vi "TP_UI.vi"() -> ()   [LabVIEW 2012]
uses:
  Global Variants/TP_GV_UI_Ref.vi
panel:
  in  "Text Ring":u16(ring)
  in  "error in":errorcluster
  in  "OK Button":bool
  out "String":string
  in  "Stop Button":bool
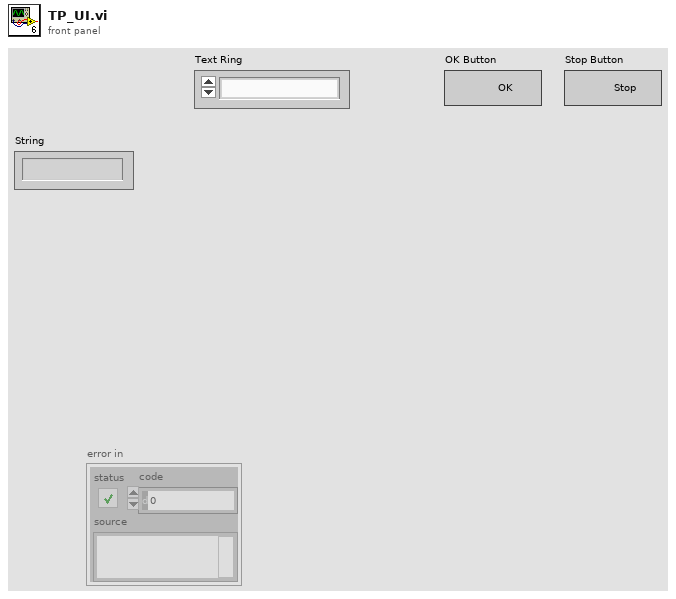
[diagram p1: front panel]
types:
  T1 = enum16{"Create Queue", "Get Queue", "Destory Queue"}
  T2 = enum16{"Create Queue", "Get Queue", "Destory Queue", "Destory all Queue"}
  T3 = cluster{"This VI":refnum<vi>, "String":refnum<vi>, "OK Button":refnum<vi>, "Stop Button":refnum<vi>, "Text Ring":refnum<vi>}
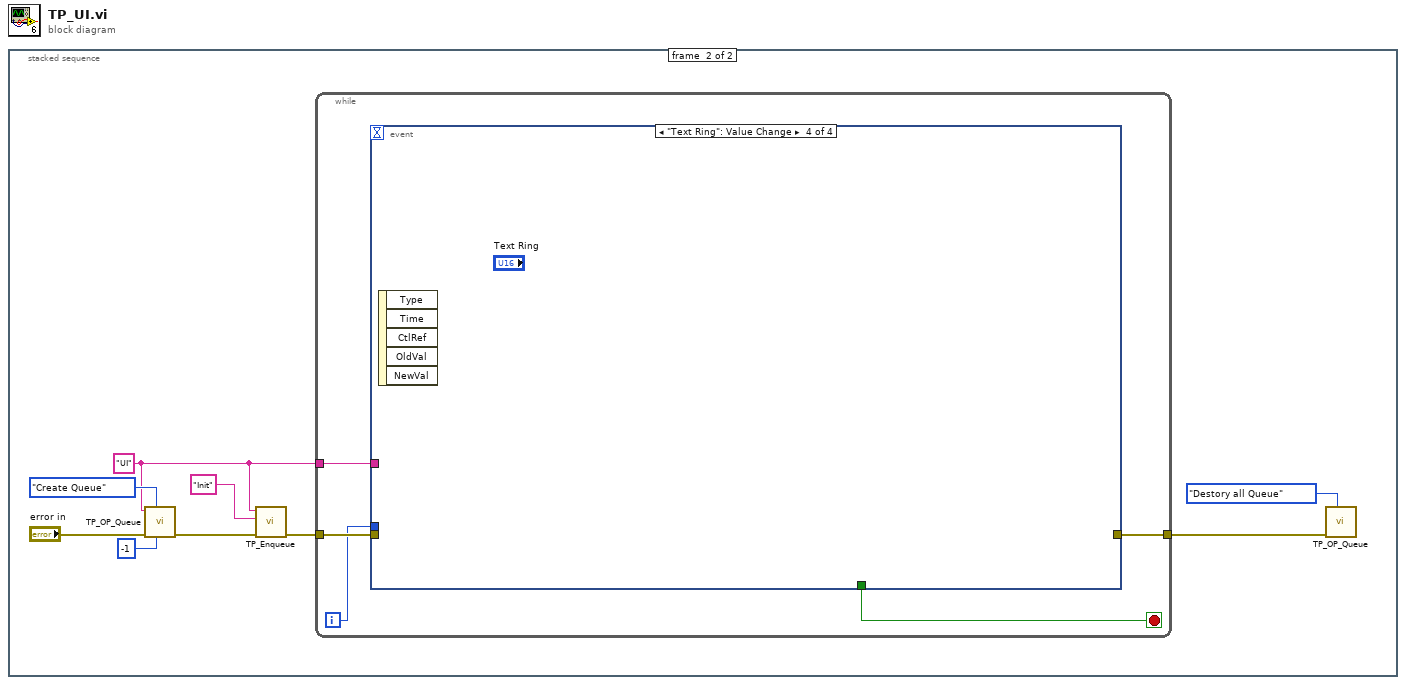
[diagram p0: block diagram]
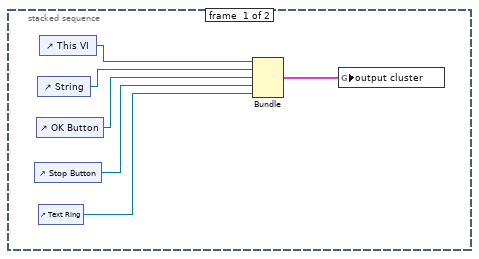
[diagram p2: hidden frame]
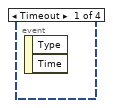
[diagram p3: hidden frame]
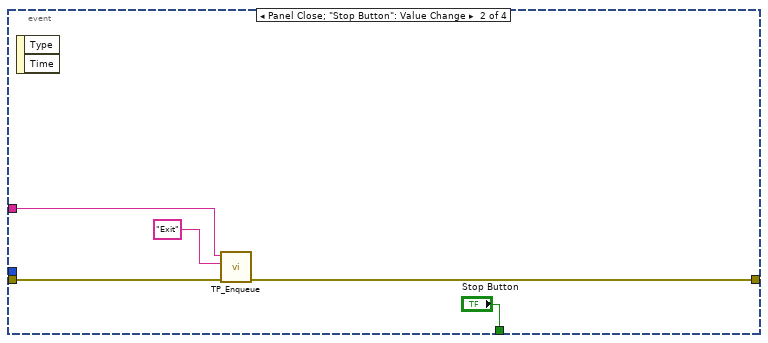
[diagram p4: hidden frame]
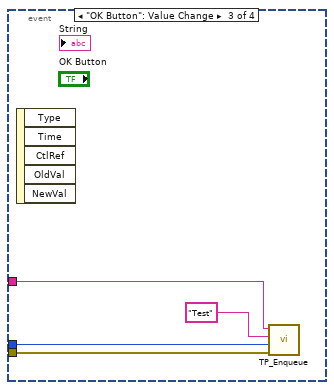
[diagram p5: hidden frame]
diagram:
  n1 = stacked-sequence {
    frame #0 {
      n2 = control-ref of="Stop Button"() -> (w3:refnum<vi>)
      n3 = control-ref of="OK Button"() -> (w4:refnum<vi>)
      n4 = control-ref of="String"() -> (w5:refnum<vi>)
      n5 = control-ref of="Text Ring"() -> (w1:refnum<vi>)
      n6 = control-ref of="This VI"() -> (w6:refnum<vi>)
      n7 = Bundle("This VI"=w6, "String"=w5, "OK Button"=w4, "Stop Button"=w3, "Text Ring"=w1) -> (w2:T3)  [unwired: 1 in]
      n8 = global write "TP_GV_UI_Ref.vi" "output cluster"(w2) -> ()
    }
    frame #1 {
      w8 = "UI" ("name (unnamed)")
      n9 = call "TP_OP_Queue.vi"("max queue size (-1, unlimited)"=-1, "OP_Queue (get queue)"=T1."Create Queue", "error in"="error in", "name (unnamed)"=w8) -> ("error out"=w9:errorcluster)  [unwired: 6 in, 1 out]
      n10 = call "TP_Enqueue.vi"("error in"=w9, "CMD"="Init", "name"=w8) -> ("error out"=w10:errorcluster)  [unwired: 8 in]
      n11 = while {
        tunnel: w10 -> [w20]
        tunnel: w8 -> [w17]
        tunnel: [w16] -> w7
        i -> [w19]
        stop <- w18 stop-if-true
        n12 = event shown="[3] \"Text Ring\": Value Change" {
          selector: _ -> [_ _ _ _]
          dyn-events: _ -> [_ _ _ _]
          timeout: _ -> [_ _ _ _]
          tunnel: w20 -> [_ w24 w29 _]
          tunnel: [_ "Stop Button" _ _] -> w18
          tunnel: w19 -> [_ _ w26 _]
          tunnel: w17 -> [_ w23 w27 _]
          tunnel: [_ w21 _ _] -> w16
          event Timeout {
            n13 = event-data() -> ()  [unwired: 1 in, 2 out]
          }
          event Panel Close; "Stop Button": Value Change {
            n14 = event-data() -> ()  [unwired: 1 in, 2 out]
            n15 = call "TP_Enqueue.vi"("error in"=w24, "CMD"="Exit", "name"=w23) -> ("error out"=w21:errorcluster)  [unwired: 8 in]
          }
          event "OK Button": Value Change {
            n16 = event-data() -> ()  [unwired: 1 in, 5 out]
            n17 = call "TP_Enqueue.vi"("error in"=w29, "Paras"=w26, "CMD"="Test" ("Message"), "name"=w27) -> ()  [unwired: 7 in, 1 out]
          }
          event "Text Ring": Value Change {
            n18 = event-data() -> ()  [unwired: 1 in, 5 out]
          }
        }
      }
      n19 = call "TP_OP_Queue.vi"("OP_Queue (get queue)"=T2."Destory all Queue", "error in"=w7) -> ()  [unwired: 8 in, 2 out]
    }
  }
